vi "Test Git Macro.vi"() -> ()   [LabVIEW 2019, in "Git.lvclass"]
uses:
  Git.lvclass
panel:
  in  "VIPB file":path
  in  "stop":bool
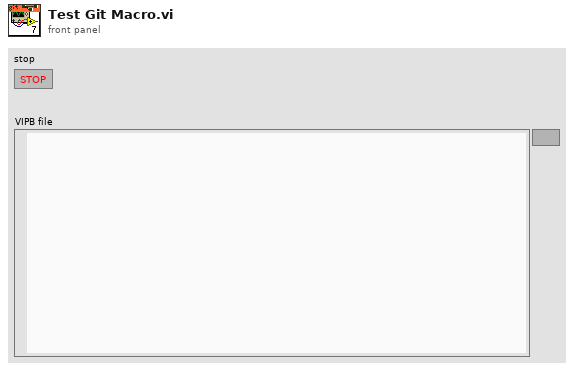
[diagram p1: front panel]
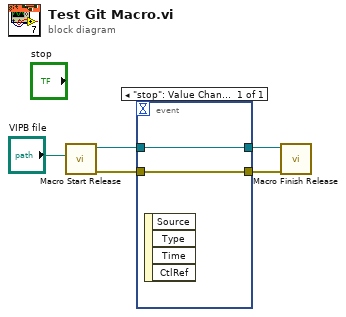
[diagram p0: block diagram]
diagram:
  n1 = call "Macro Start Release.vi"("VIPB Path"="VIPB file") -> ("error out"=w3:errorcluster, "Git out"=w5:refnum<class "Git.lvclass">)  [unwired: 9 in]
  n2 = event shown="[0] \"stop\": Value Change" {
    selector: _ -> [_]
    dyn-events: _ -> [_]
    timeout: _ -> [_]
    tunnel: w5 -> [w6]
    tunnel: [w7] -> w4
    tunnel: w3 -> [w7]
    tunnel: [w6] -> w2
    event "stop": Value Change {
      n3 = event-data() -> ()  [unwired: 1 in, 4 out]
    }
  }
  n4 = call "Macro Finish Release.vi"("error in (no error)"=w4, "Git in"=w2) -> ()  [unwired: 7 in, 3 out]
